vi "Set Zero Mode.vi"(8 "error in (no error)":errorcluster, 9 "Firmware Revision":string(combo), 10 "zero mode (F)":bool, 11 "VISA resource name":refnum<visa-resource-name>) -> (0 "error out":errorcluster, 1 "measurement results":T2, 2 "bridge error":T1, 3 "VISA resource name out":refnum<visa-resource-name>)   [LabVIEW 2019, in "Andeen-Hagerling 2700A.lvlib"]
doc: "Enables or disables the Zero compensation result mode.\nWhen enabled, the Zero compensation result mode compensates\nfor residual capacitance and parallel loss effects that\nare usually inherent in test fixtures."
uses:
  Andeen-Hagerling 2700A.lvlib
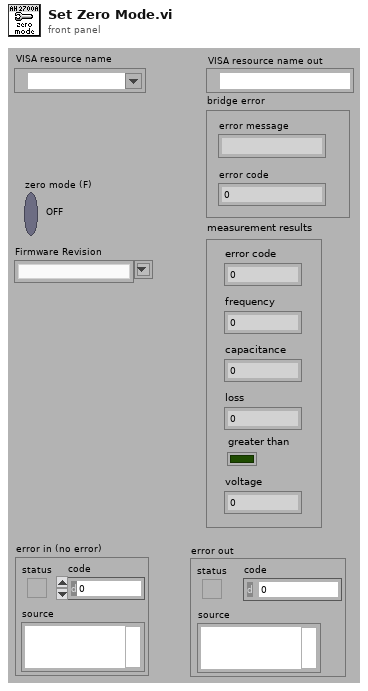
[diagram p1: front panel]
types:
  T1 = cluster{"error message":string, "error code":i32}
  T2 = cluster{"error code":i32, "frequency":dbl, "capacitance":dbl, "loss":dbl, "greater than":bool, "voltage":dbl}
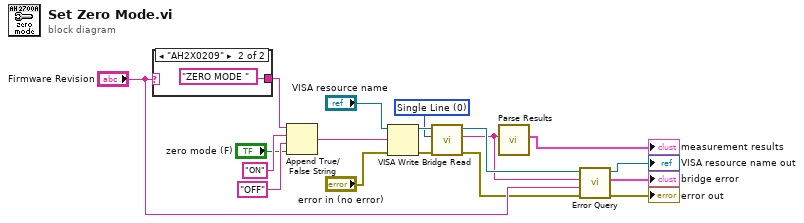
[diagram p0: block diagram]
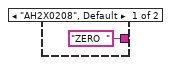
[diagram p2: hidden frame]
diagram:
  w1 = u16 0 items=["Single Line", "Multi-Line"] ("Multiline")
  n1 = case shown="\"AH2X0209\"" "Firmware Revision" {
    tunnel: ["ZERO  " "ZERO MODE "] -> w12
    frame "AH2X0208", Default {
    }
    frame "AH2X0209" {
    }
  }
  n2 = Append True/False String(1:"zero mode (F)", 2:"OFF" ("false string"), 3:"ON" ("true string"), 4:w12) -> (0:w14:string)
  n3 = VISA Write(VISA resource name="VISA resource name", write buffer=w14, error in (no error)="error in (no error)") -> (VISA resource name out=w6:refnum<visa-resource-name>, error out=w5:errorcluster)  [unwired: 1 out]
  n4 = call "Bridge Read.vi"("error in (no error)"=w5, "multiline"=w1, "VISA resource name"=w6) -> ("error out"=w4:errorcluster, "read buffer"=w2:string, "VISA resource name out"=w3:refnum<visa-resource-name>)  [unwired: 6 in]
  n5 = call "Parse Results.vi"("measurement line"=w2) -> ("measurement results"=→"measurement results":T2)  [unwired: 9 in]
  n6 = call "Error Query.vi"("error in (no error)"=w4, "firmware revision"="Firmware Revision", "measurement line"=w2, "VISA resource name"=w3) -> ("error out"=→"error out":errorcluster, "bridge error"=→"bridge error":T1, "VISA resource name out"=→"VISA resource name out":refnum<visa-resource-name>)  [unwired: 5 in]
